vi "fileLoadFloatArray.vi"(11 "File Path":path=path "c:/bob.dat") -> (3 "output array":dbl[][](array[numeric]))   [LabVIEW 2010, in "kevLib2010.lvlib"]
uses:
  kevLib2010.lvlib
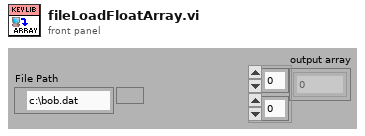
[diagram p1: front panel]
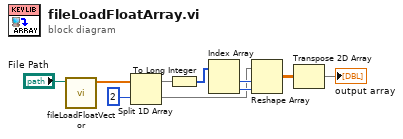
[diagram p0: block diagram]
diagram:
  n1 = call "fileLoadFloatVector.vi"("File Path"="File Path") -> ("Float Vector"=w10:dbl[])  [unwired: 9 in, 1 out]
  n2 = Split 1D Array(array=w10, index=2) -> (first subarray=w8:dbl[], second subarray=w4:dbl[])
  n3 = To Long Integer(number=w8) -> (32bit integer=w7:i32[])
  n4 = Index Array(array=w7) -> (element #1=w6:i32, element #2=w5:i32)  [unwired: 2 in]
  n5 = Reshape Array(w4, w6, w5) -> (w2:dbl[][])
  n6 = Transpose 2D Array(2D array=w2) -> (transposed array=→"output array":dbl[][])
